vi "Builder.Set Framework Cache.vi"(10 "Framework Cache":refnum<class "DSF.Engine.Memory.Cache.Framework.lvclass">, 11 "Builder in":refnum<class "Builder.lvclass">) -> (3 "Builder out":refnum<class "Builder.lvclass">)   [LabVIEW 2016, in "DSF.Engine.lvlib" / "Builder.lvclass"]
uses:
  Builder.lvclass
  Cache/DSF.Engine.Memory.Cache.Framework.lvclass
  Builder.lvclass/Builder.ctl
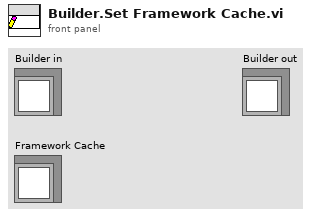
[diagram p1: front panel]
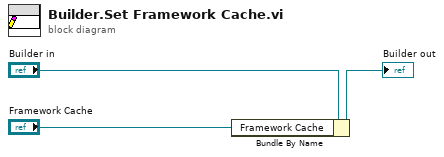
[diagram p0: block diagram]
diagram:
  n1 = Bundle By Name(cluster="Builder in", "Framework Cache"="Framework Cache") -> (→"Builder out":refnum<class "Builder.lvclass">)
